vi "subGenerateDGMLOwnerlessFilesFolderString.vi"(7 "Expand?":bool, 8 "error in (no error)":errorcluster, 9 "Links in":T1, 10 "Nodes in":T1, 11 "ILabVIEWItem in":refnum<class "ILabVIEWItem.lvclass">) -> (0 "error out":errorcluster, 1 "Links":T1, 2 "Nodes":T1, 3 "ILabVIEWItem out":refnum<class "ILabVIEWItem.lvclass">, 4 "Path":string="Z:\\OtherFiles")   [LabVIEW 2020, in "DefaultExtensions.lvlib" / "CGrapherDGML.lvclass"]
uses:
  CGrapherDGML.lvclass
  obj/Addons/LabVIEWObjectInterfaces.lvlibp/LabVIEWObjectInterfaces/ILabVIEWItem/ILabVIEWItem.lvclass
  obj/Addons/LabVIEWItem.lvlibp/LabVIEWItem/CLabVIEWItem/ConnectionSet.ctl
  ecf4d353-cf80-4459-a486-8bebc84a9ab0.vi
  obj/Addons/LabVIEWItem.lvlibp/LabVIEWItem/CLabVIEWItem/CLabVIEWItem.lvclass
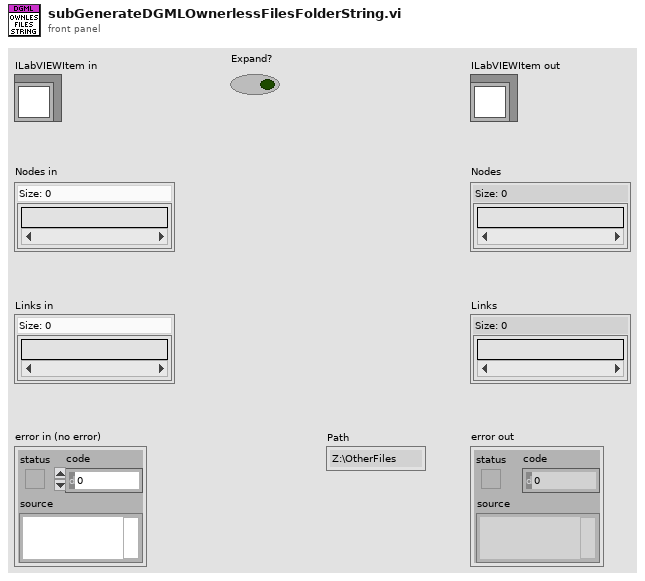
[diagram p1: front panel]
types:
  T1 = typedef "LabVIEWItem.lvlibp/CLabVIEWItem.lvclass/ConnectionSet.ctl" = set{string}
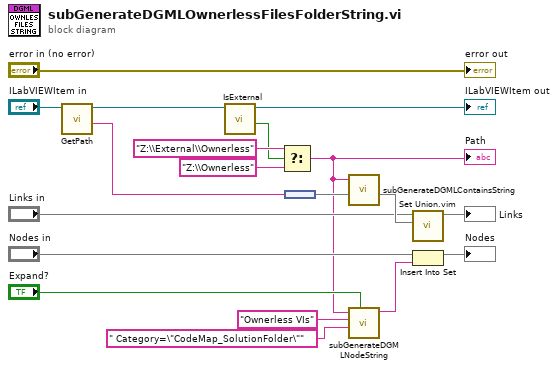
[diagram p0: block diagram]
diagram:
  n1 = call-dynamic "GetPath.vi"("ILabVIEWItem in"="ILabVIEWItem in") -> ("Path"=w18:string, "ILabVIEWItem out"=w12:refnum<class "ILabVIEWItem.lvclass">)  [unwired: 8 in, 1 out]
  n2 = call-dynamic "IsExternal.vi"("ILabVIEWItem in"=w12) -> ("Is external?"=w2:bool, "ILabVIEWItem out"=→"ILabVIEWItem out":refnum<class "ILabVIEWItem.lvclass">)  [unwired: 8 in, 1 out]
  n3 = Select(t="Z:\\External\\Ownerless" ("format string"), s=w2, f="Z:\\Ownerless" ("format string")) -> (s? t:f=w1:string)
  "Path" <- w1
  n4 = node(w18) -> (w17:set{string})
  n5 = call "subGenerateDGMLContainsString.vi"("Contained"=w17, "Source"=w1) -> ("Links"=w16:T1)  [unwired: 9 in]
  n6 = call "subGenerateDGMLNodeString.vi"("Expand?"="Expand?", "Code schema"=" Category=\"CodeMap_SolutionFolder\"" ("format string"), "Label"="Ownerless VIs" ("format string"), "Id"=w1) -> ("Node string"=w14:string)  [unwired: 7 in]
  n7 = call "Set Union.vim"("set 2"=w16, "set 1"="Links in") -> ("union"=→"Links":T1)  [unwired: 9 in]
  n8 = Insert Into Set(10:w14, 11:"Nodes in") -> (3:→"Nodes":T1)  [unwired: 1 out]
  "error out" <- "error in (no error)"
